vi "Initialize Soft Limits.vi"(8 "error in (no error)":errorcluster, 11 "Port In":T1={"P type"=0, "reference"="", " Terminator "="\r\n", "Timeout"=300} {"Timeout" step=10; "P type" items=["none", "RS-232C"]}) -> (0 "error out":errorcluster, 3 "Port Out":T1={"P type"=0, "reference"="", " Terminator "="\r\n", "Timeout"=300} {"Timeout" step=10; "P type" items=["none", "RS-232C"]})   [LabVIEW 2021]
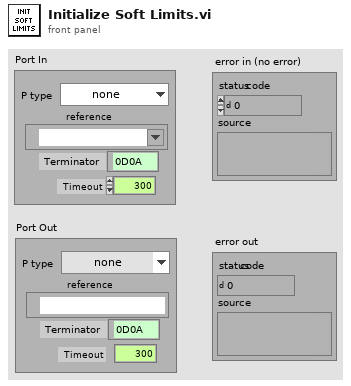
[diagram p1: front panel]
types:
  T1 = cluster{"P type":u16, "reference":refnum<visa-resource-name>, " Terminator ":string, "Timeout":i32}
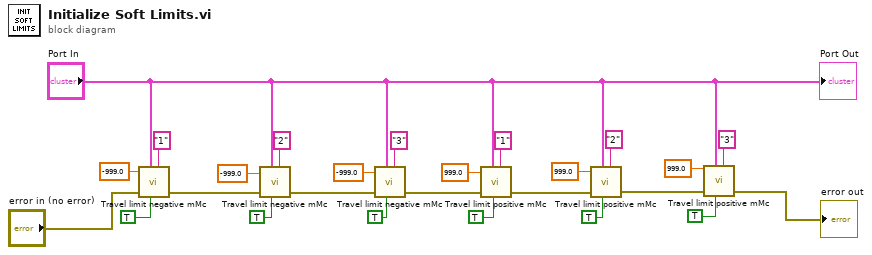
[diagram p0: block diagram]
diagram:
  n1 = call "Travel limit negative mMc.vi"("limit in"=-999.0, "Port"="Port In", "error in (no error)"="error in (no error)", "set/get"=TRUE, "Controller #"="1") -> ("error out"=w16:errorcluster)  [unwired: 3 in, 1 out]
  n2 = call "Travel limit negative mMc.vi"("limit in"=-999.0, "Port"="Port In", "error in (no error)"=w16, "set/get"=TRUE, "Controller #"="2") -> ("error out"=w17:errorcluster)  [unwired: 3 in, 1 out]
  n3 = call "Travel limit negative mMc.vi"("limit in"=-999.0, "Port"="Port In", "error in (no error)"=w17, "set/get"=TRUE, "Controller #"="3") -> ("error out"=w18:errorcluster)  [unwired: 3 in, 1 out]
  n4 = call "Travel limit positive mMc.vi"("limit in"=999.0, "Port"="Port In", "error in (no error)"=w18, "set/get"=TRUE, "Controller #"="1") -> ("error out"=w19:errorcluster)  [unwired: 3 in, 1 out]
  n5 = call "Travel limit positive mMc.vi"("limit in"=999.0, "Port"="Port In", "error in (no error)"=w19, "set/get"=TRUE, "Controller #"="2") -> ("error out"=w20:errorcluster)  [unwired: 3 in, 1 out]
  n6 = call "Travel limit positive mMc.vi"("limit in"=999.0, "Port"="Port In", "error in (no error)"=w20, "set/get"=TRUE, "Controller #"="3") -> ("error out"=→"error out":errorcluster)  [unwired: 3 in, 1 out]
  "Port Out" <- "Port In"
